vi "shift.vi"(9 "Setting":path=path "D:/data/Test Settings") -> (2 "data":T1 {"Shift-C" format="%<%H:%M>T"; "Shift-B" format="%<%H:%M>T"; "Shift-A" format="%<%H:%M>T"}, 3 "SHIFT_A":string)   [LabVIEW 2023]
uses:
  Controls/Communication setting.ctl
panel:
  out "error out":errorcluster
  out "B":bool
  out "A":bool
  out "x+y 4":i32
  out "x+y 3":i32
  out "x+y 2":i32
  out "x+y":i32
  out "Minutes":string
  out "Hour":string
  out "date time rec":T2
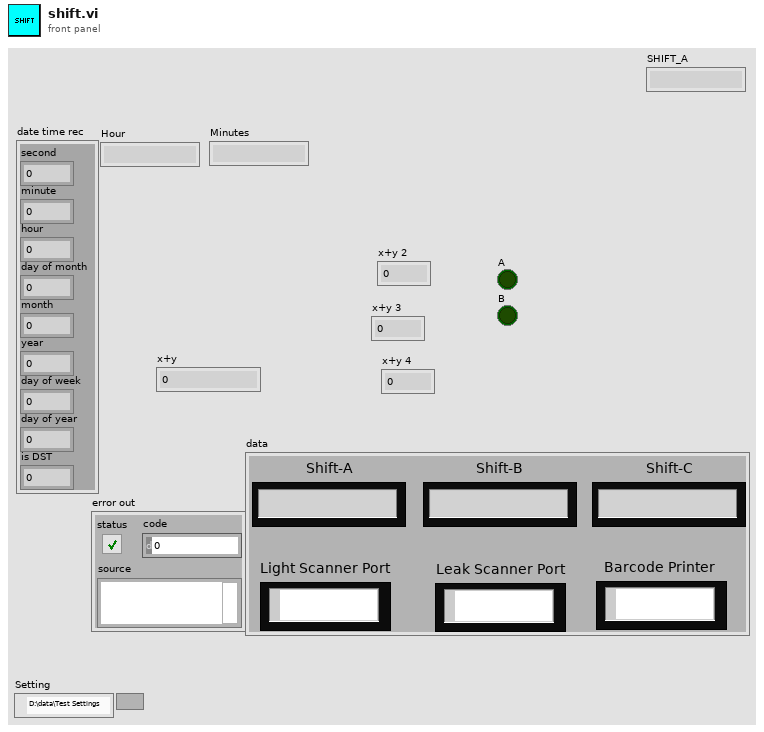
[diagram p1: front panel]
types:
  T1 = typedef "Communication setting.ctl" = cluster{"Light Scanner Port":refnum<visa-resource-name>, "Shift-A":timestamp, "Shift-B":timestamp, "Shift-C":timestamp, "Leak Scanner Port":refnum<visa-resource-name>, "Barcode Printer":refnum<visa-resource-name>}
  T2 = cluster{"second":i32, "minute":i32, "hour":i32, "day of month":i32, "month":i32, "year":i32, "day of week":i32, "day of year":i32, "is DST":i32}
  T3 = cluster{"Shift-A":timestamp, "Shift-A":timestamp, "Shift-A":timestamp, "Printer Port":refnum<visa-resource-name>}
  T4 = enum16{"open", "replace", "create", "open or create", "replace or create", "replace or create with confirmation"}
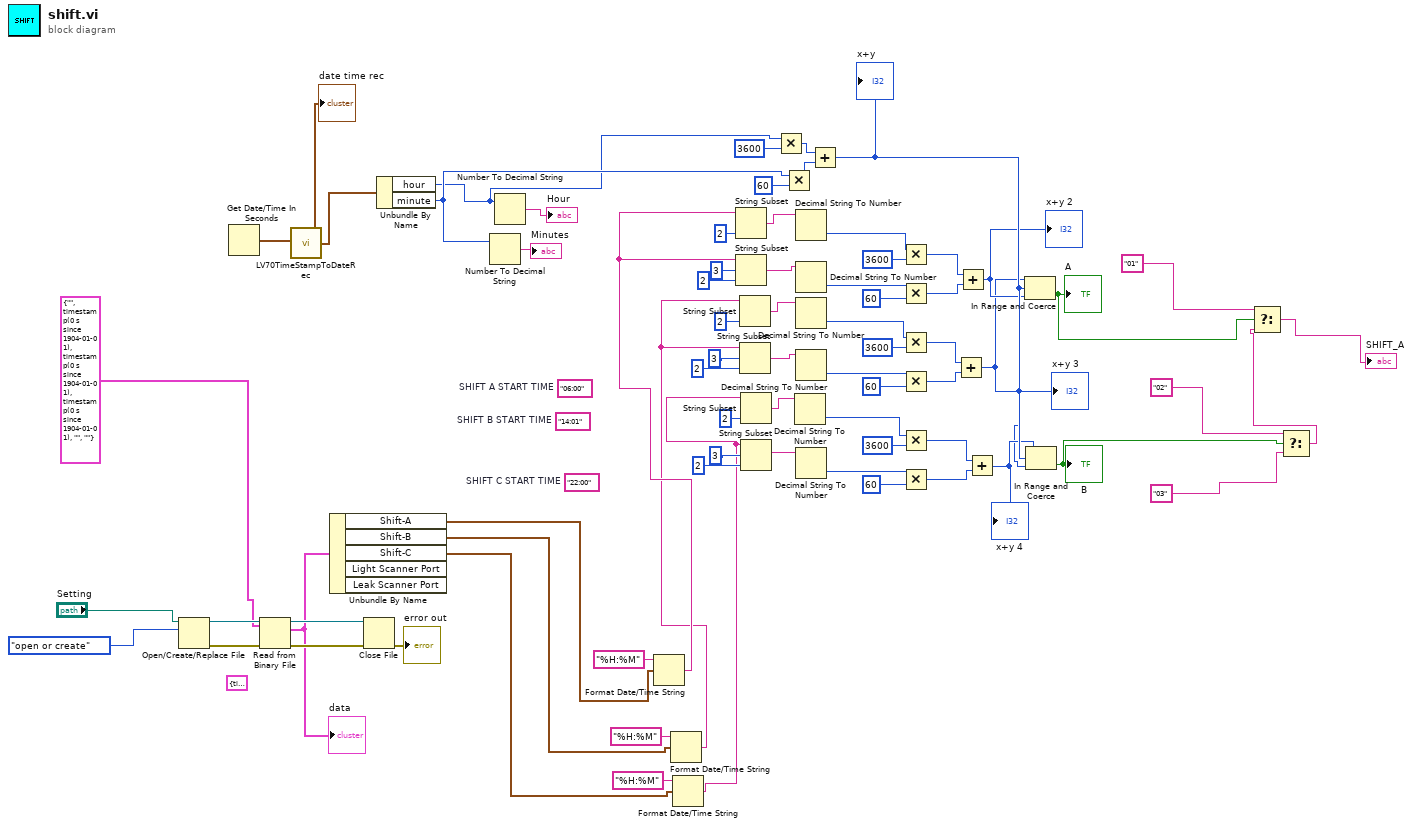
[diagram p0: block diagram]
diagram:
  (unwired) T3 {"Shift-A"=timestamp(0 s since 1904-01-01), "Shift-A"=timestamp(0 s since 1904-01-01), "Shift-A"=timestamp(0 s since 1904-01-01), "Printer Port"=""} ("output cluster")
  (unwired) "22:00"  # SHIFT C START TIME
  (unwired) "14:01"  # SHIFT B START TIME
  (unwired) "06:00"  # SHIFT A START TIME
  n1 = Open/Create/Replace File(file path (use dialog)="Setting", operation (0:open)=T4."open or create") -> (refnum out=w11:refnum<file>, error out=w12:errorcluster)  [unwired: 4 in, 1 out]
  n2 = Get Date/Time In Seconds() -> (seconds since 1Jan1904=w72:timestamp)
  n3 = Read from Binary File(5:T1 {"Light Scanner Port"="", "Shift-A"=timestamp(0 s since 1904-01-01), "Shift-B"=timestamp(0 s since 1904-01-01), "Shift-C"=timestamp(0 s since 1904-01-01), "Leak Scanner Port"="", "Barcode Printer"=""} ("output cluster"), 8:w12, 11:w11) -> (0:w9:errorcluster, 2:w8:T1, 3:w10:refnum<file>)  [unwired: 3 in, 1 out]
  "data" <- w8
  n4 = call <vilib>:"LV70TimeStampToDateRec.vi"("time stamp"=w72) -> ("date time rec"=w71:T2)
  "date time rec" <- w71
  n5 = Unbundle By Name(w8) -> ("Shift-A"=w7:timestamp, "Shift-B"=w6:timestamp, "Shift-C"=w5:timestamp)  [unwired: 2 out]
  n6 = Close File(refnum=w10, error in=w9) -> (error out=→"error out":errorcluster)  [unwired: 1 out]
  n7 = Unbundle By Name(w71) -> ("hour"=w28:i32, "minute"=w59:i32)
  n8 = Number To Decimal String(number=w59) -> (decimal integer string=→"Minutes":string)  [unwired: 1 out]
  n9 = Number To Decimal String(number=w28) -> (decimal integer string=→"Hour":string)  [unwired: 1 out]
  n10 = Format Date/Time String(time format string (%c)="%H:%M", seconds (now)=w7) -> (date/time string=w15:string)  [unwired: 1 in]
  n11 = Format Date/Time String(time format string (%c)="%H:%M", seconds (now)=w6) -> (date/time string=w14:string)  [unwired: 1 in]
  n12 = Format Date/Time String(time format string (%c)="%H:%M", seconds (now)=w5) -> (date/time string=w13:string)  [unwired: 1 in]
  n13 = String Subset(string=w15, length (rest)=2 ("length (rest)")) -> (substring=w58:string)  [unwired: 1 out]
  n14 = String Subset(string=w15, offset (0)=3 ("length (rest)"), length (rest)=2 ("length (rest)")) -> (substring=w54:string)
  n15 = String Subset(string=w14, length (rest)=2 ("length (rest)")) -> (substring=w36:string)  [unwired: 1 out]
  n16 = String Subset(string=w14, offset (0)=3 ("length (rest)"), length (rest)=2 ("length (rest)")) -> (substring=w35:string)
  n17 = String Subset(string=w13, length (rest)=2 ("length (rest)")) -> (substring=w45:string)  [unwired: 1 out]
  n18 = String Subset(string=w13, offset (0)=3 ("length (rest)"), length (rest)=2 ("length (rest)")) -> (substring=w44:string)
  n19 = Multiply(x=w28, y=3600) -> (x*y=w31:i32)
  n20 = Multiply(x=w59, y=60) -> (x*y=w30:i32)
  n21 = Decimal String To Number(string=w45) -> (number=w46:i32)  [unwired: 3 out]
  n22 = Decimal String To Number(string=w58) -> (number=w57:i32)  [unwired: 3 out]
  n23 = Decimal String To Number(string=w54) -> (number=w53:i32)  [unwired: 3 out]
  n24 = Decimal String To Number(string=w36) -> (number=w37:i32)  [unwired: 3 out]
  n25 = Decimal String To Number(string=w35) -> (number=w40:i32)  [unwired: 3 out]
  n26 = Decimal String To Number(string=w44) -> (number=w48:i32)  [unwired: 3 out]
  n27 = Add(x=w31, y=w30) -> (x+y=w34:i32)
  "x+y" <- w34
  n28 = Multiply(x=w57, y=3600) -> (x*y=w52:i32)
  n29 = Multiply(x=w53, y=60) -> (x*y=w51:i32)
  n30 = Multiply(x=w37, y=3600) -> (x*y=w41:i32)
  n31 = Multiply(x=w40, y=60) -> (x*y=w42:i32)
  n32 = Multiply(x=w46, y=3600) -> (x*y=w49:i32)
  n33 = Multiply(x=w48, y=60) -> (x*y=w50:i32)
  n34 = Add(x=w41, y=w42) -> (x+y=w26:i32)
  "x+y 3" <- w26
  n35 = Add(x=w52, y=w51) -> (x+y=w29:i32)
  "x+y 2" <- w29
  n36 = Add(x=w49, y=w50) -> (x+y=w27:i32)
  "x+y 4" <- w27
  n37 = In Range and Coerce(upper limit=w26, x=w34, lower limit=w29) -> (In Range?=w25:bool)  [unwired: 1 out]
  "A" <- w25
  n38 = In Range and Coerce(upper limit=w27, x=w34, lower limit=w26) -> (In Range?=w22:bool)  [unwired: 1 out]
  "B" <- w22
  n39 = Select(t="02", s=w22, f="03") -> (s? t:f=w20:string)
  n40 = Select(t="01", s=w25, f=w20) -> (s? t:f=→"SHIFT_A":string)
